vi "_Serial Port-Clear_Receive_Buffer.vi"(5 "Serial Port":refnum<visa-resource-name>="COM5") -> (0 "error out":errorcluster, 2 "Serial Port out":refnum<visa-resource-name>="COM5")   [LabVIEW 2015]
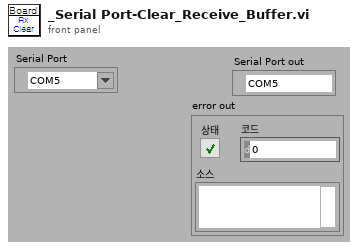
[diagram p1: front panel]
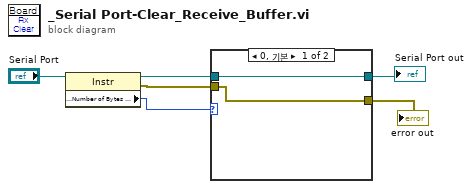
[diagram p0: block diagram]
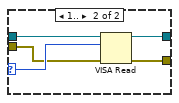
[diagram p2: hidden frame]
diagram:
  n1 = property class="Instr"(reference="Serial Port") -> (reference out=w6:refnum<visa-resource-name>, error out=w2:errorcluster, "Serial Settings:Number of Bytes at Serial Port"=w3:u32)  [unwired: 1 in]
  n2 = case shown="0, 기본" w3 {
    selector: w3 -> [_ w11]
    tunnel: w6 -> [w8 w13]
    tunnel: [w8 w12] -> w4
    tunnel: w2 -> [w7 w10]
    tunnel: [w7 w9] -> w1
    frame 0, Default {
    }
    frame 1.. {
      n3 = VISA Read(VISA resource name=w13, byte count=w11, error in (no error)=w10) -> (VISA resource name out=w12:refnum<visa-resource-name>, error out=w9:errorcluster)  [unwired: 2 out]
    }
  }
  "Serial Port out" <- w4
  "error out" <- w1
